vi "DAQ Engine Edit.vi"(8 "error in":errorcluster, 10 "DAQ Engine":string(combo), 11 "Sequence Context In":refnum<k7>) -> (0 "error out":errorcluster, 3 "DAQ Engine Out":string(combo))   [LabVIEW 2023, in "LTT_TeststandSteptypes.lvlib"]
uses:
  LTT_TeststandSteptypes.lvlib
  <vilib>/addons/TestStand/_TSUtility.llb/TestStand - Start Modal Dialog (Sequence Context).vi
  <vilib>/addons/TestStand/_TSUtility.llb/TestStand - End Modal Dialog (Sequence Context).vi
  HardwareAbstractionLayer_LVOOP/Database/Database.lvclass
  HardwareAbstractionLayer_LVOOP/Database/SQL Public VI/Control/DB Options.ctl
panel:
  in  "Close":bool
  in  "OK":bool
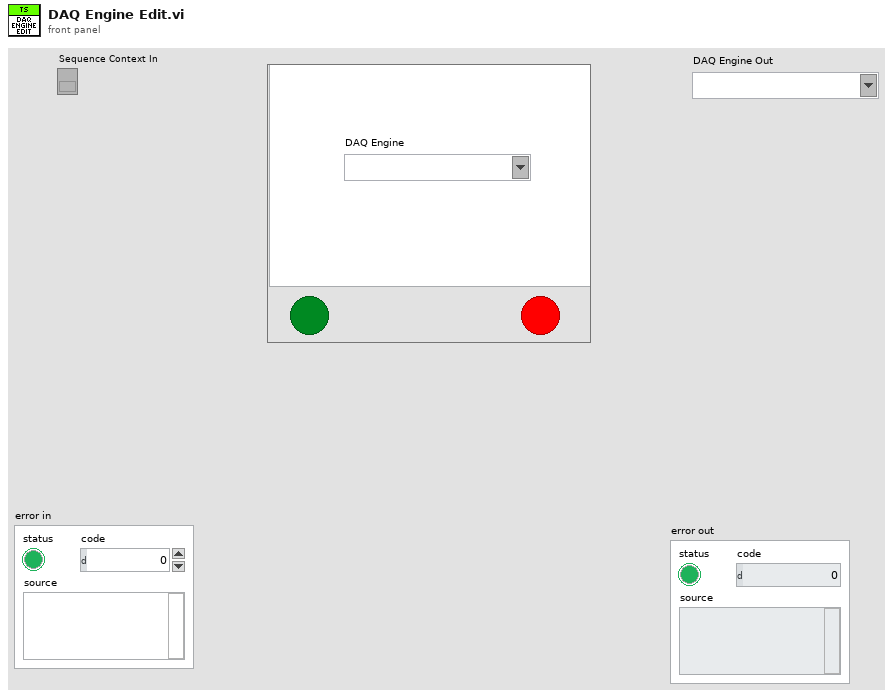
[diagram p1: front panel]
types:
  T1 = typedef "HardwareAbstractionLayer_LVOOP.lvlib/Database.lvclass/DB Options.ctl" = enum16{"Init", "Select Data", "Insert Data", "Update Data", "Delete Data", "Execute Query", "Create Schema", "Create Table", "List Tables", "List Columns", "Close"}
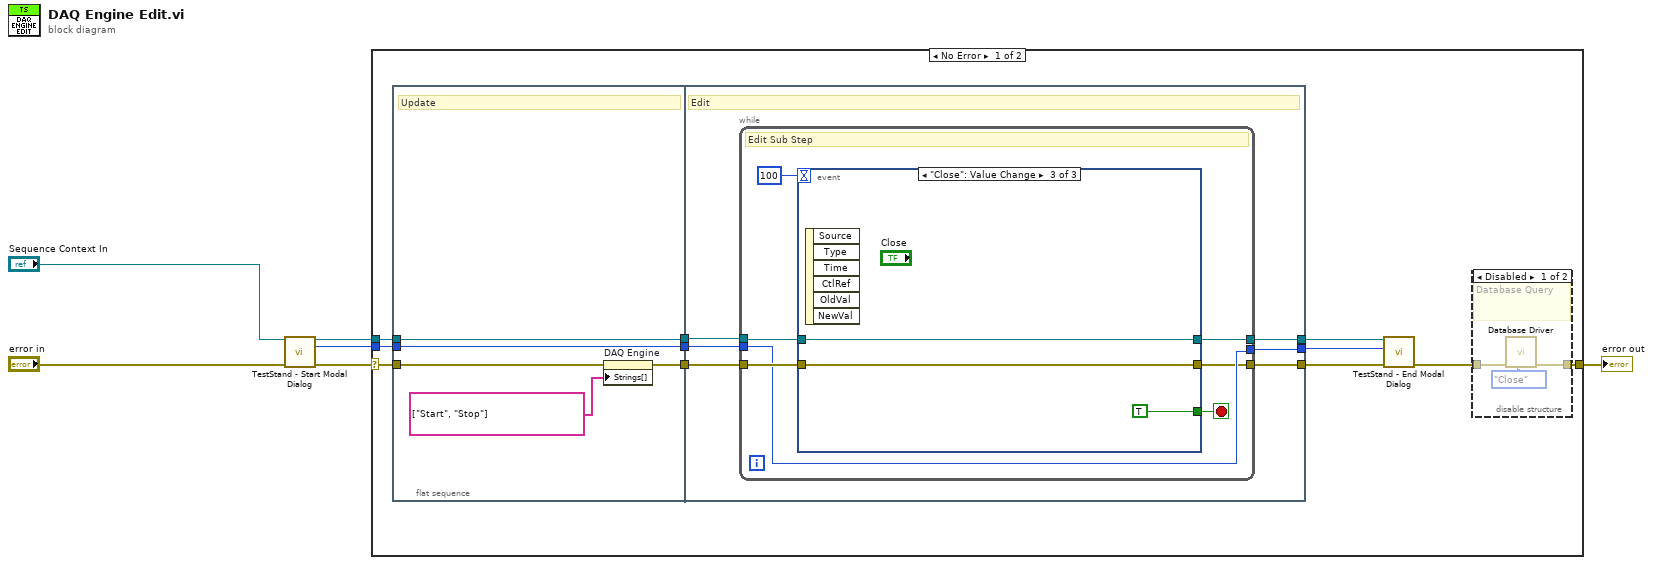
[diagram p0: block diagram]
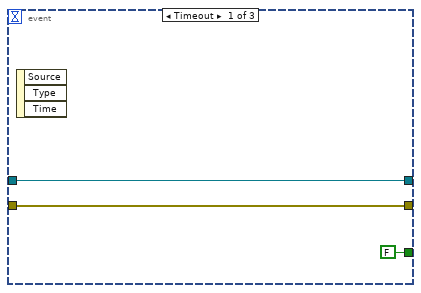
[diagram p3: hidden frame]
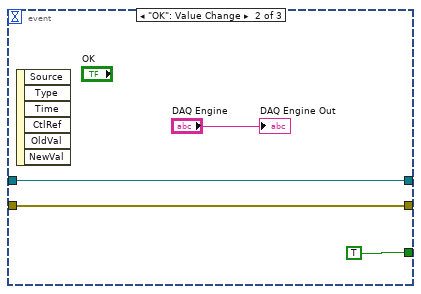
[diagram p4: hidden frame]
diagram:
  n1 = call-poly <vilib>:"TestStand - Start Modal Dialog.vi"("Sequence Context In"="Sequence Context In", "error in (no error)"="error in") -> ("Sequence Context Out"=w4:refnum<k7>, "Modal ID"=w3:i32, "error out"=w5:errorcluster)  [unwired: 9 in, 2 out]
  n2 = case shown="No Error" w5 {
    selector: w5 -> [w14 w49]
    tunnel: w4 -> [w11 _]
    tunnel: w3 -> [w10 _]
    tunnel: [w7 w49] -> w2
    frame No Error {
      n3 = flat-sequence {
        tunnel: w14 -> [w22]
        tunnel: [w21] -> w17
        tunnel: w11 -> [w25]
        tunnel: w10 -> [w24]
        tunnel: [w25] -> w16
        tunnel: [w24] -> w15
        tunnel: w17 -> [w29]
        tunnel: [w27] -> w13
        tunnel: w16 -> [w31]
        tunnel: w15 -> [w30]
        tunnel: [w28] -> w9
        tunnel: [w26] -> w8
        frame #0 {
          # "Update"
          n4 = property on="DAQ Engine" class="CmbBox"(error in=w22, "Strings[]"=string[] ["Start", "Stop"] ("Strings []")) -> (error out=w21:errorcluster)  [unwired: 1 in, 1 out]
        }
        frame #1 {
          # "Edit"
          n5 = while {
            tunnel: w31 -> [w36]
            tunnel: w30 -> [w33]
            tunnel: w29 -> [w34]
            tunnel: [w35] -> w26
            tunnel: [w33] -> w28
            tunnel: [w32] -> w27
            stop <- w37 stop-if-true
            # "Edit Sub Step"
            n6 = event shown="[2] \"Close\": Value Change" {
              selector: _ -> [_ _ _]
              dyn-events: _ -> [_ _ _]
              timeout: 100 -> [_ _ _]
              tunnel: [FALSE TRUE TRUE] -> w37
              tunnel: [w41 w42 w47] -> w35
              tunnel: w36 -> [w41 w42 w47]
              tunnel: w34 -> [w40 w43 w46]
              tunnel: [w40 w43 w46] -> w32
              event Timeout {
                n7 = event-data() -> ()  [unwired: 1 in, 3 out]
              }
              event "OK": Value Change {
                n8 = event-data() -> ()  [unwired: 1 in, 6 out]
                "DAQ Engine Out" <- "DAQ Engine"
              }
              event "Close": Value Change {
                n9 = event-data() -> ()  [unwired: 1 in, 6 out]
              }
            }
          }
        }
      }
      n10 = call-poly <vilib>:"TestStand - End Modal Dialog.vi"("Sequence Context In"=w8, "Modal ID"=w9, "error in (no error)"=w13) -> ("error out"=w12:errorcluster)  [unwired: 12 in]
      n11 = disable-structure shown="Disabled" {
        disable-tunnel: w12 -> [w20 _]
        disable-tunnel: [w19 _] -> w7
        frame Disabled {
          # "Need to Enable for Database Query"
          n12 = call "Database Driver.vi"("Options"=DB_Options."Close", "error in"=w20) -> ("error out"=w19:errorcluster)  [unwired: 6 in, 3 out]
        }
        frame Enabled {
        }
      }
    }
    frame Error {
    }
  }
  "error out" <- w2
